vi "Get Starting Context.vi"(8 "error in (no error)":errorcluster, 11 "Search in":refnum<class "Search.lvclass">) -> (0 "error out":errorcluster, 2 "Starting Context":T1, 3 "Search out":refnum<class "Search.lvclass">)   [LabVIEW 2020, in "Better Search.lvlib" / "Search.lvclass"]
uses:
  Search.lvclass
  Data Types/Search Context.ctl
  Data Types/Start Search Type.ctl
  Data Types/Type Reflection Item.ctl
  Search.lvclass/Search.ctl
  Better Search.lvlib
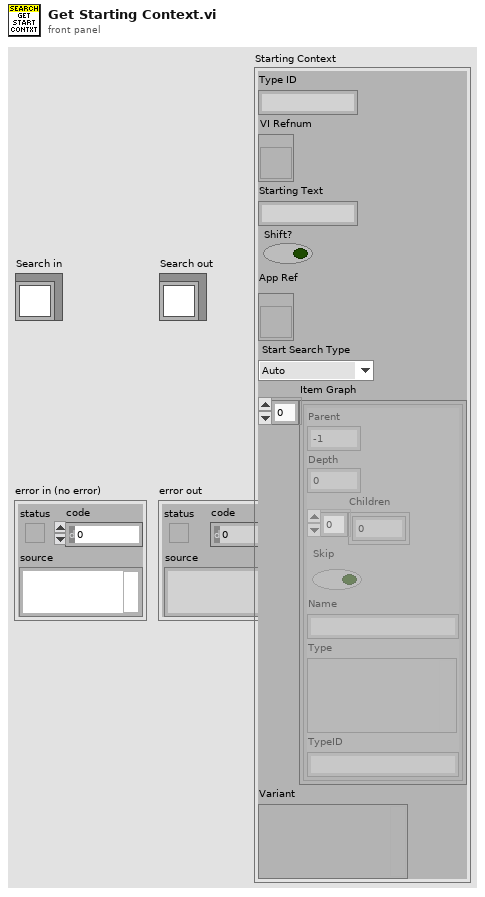
[diagram p1: front panel]
types:
  T1 = typedef "Better Search.lvlib/Search Context.ctl" = cluster{"Type ID":string, "VI Refnum":refnum<vi>, "Starting Text":string, "Shift?":bool, "App Ref":refnum<vi>, "Start Search Type":T2, "Item Graph":T3[], "Variant":variant}
  T2 = typedef "Better Search.lvlib/Start Search Type.ctl" = enum16{"Auto", "Text", "Data Type", "Bundle"}
  T3 = typedef "Better Search.lvlib/Type Reflection Item.ctl" = cluster{"Parent":i32, "Depth":i32, "Children":i32[], "Skip":bool, "Name":string, "Type":variant, "TypeID":string}
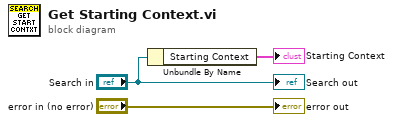
[diagram p0: block diagram]
diagram:
  n1 = Unbundle By Name("Search in") -> ("Starting Context"=→"Starting Context":T1)
  "error out" <- "error in (no error)"
  "Search out" <- "Search in"
